vi "SV Compute Statistical Level from Waveform.vi"(0 "waveform data":waveform(dbl), 5 "N (50 %)":dbl=50.0 min=0.0 max=100.0 step=0.5) -> (4 "sorted data":dbl[](array[numeric]), 6 "L_N":dbl=nan min=0.0 max=100.0 step=0.5 format="%_4g")   [LabVIEW 2017]
doc: "Use this VI to return <B>L_N</B> levels where L_N is the level which N % of the values exceed. For example, L50 represents the median, where 50 % of the values are greater than L_N and 50 % are lower. L90 is commonly used as a noise baseline, as 90 % of the values exceed L_N. L10 is commonly used as a measure of peak levels because it corresponds to the highest 10 % of levels."
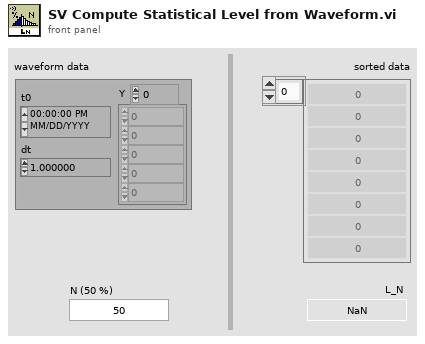
[diagram p1: front panel]
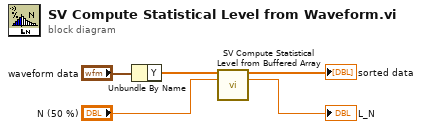
[diagram p0: block diagram]
diagram:
  n1 = Unbundle By Name("waveform data") -> ("Y"=w4:dbl[])
  n2 = call <vilib>:"SV Compute Statistical Level from Buffered Array.vi"("data"=w4, "N (50 %)"="N (50 %)") -> ("sorted data"=→"sorted data":dbl[], "L_N"=→"L_N":dbl)  [unwired: 12 in]
